vi "Reset Merlin SLM.vi"   [LabVIEW 2014]
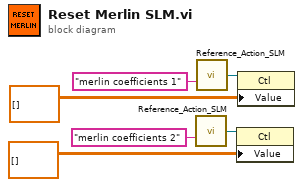
[diagram p0: block diagram]
diagram:
  n1 = call "Reference_Action_SLM.vi"("Control Name"="merlin coefficients 2") -> ("Ref OUT"=w2:refnum<vi>)  [unwired: 12 in, 2 out]
  n2 = call "Reference_Action_SLM.vi"("Control Name"="merlin coefficients 1") -> ("Ref OUT"=w5:refnum<vi>)  [unwired: 12 in, 2 out]
  n3 = property class="Ctl"(reference=w2, "Value"=dbl[][] [] ("Mode Coeffs")) -> ()  [unwired: 1 in, 2 out]
  n4 = property class="Ctl"(reference=w5, "Value"=dbl[][] [] ("Mode Coeffs")) -> ()  [unwired: 1 in, 2 out]
